vi "MotorControllerOpen.vi"(3 "error in":errorcluster, 4 "RefnumName":string, 5 "MotorConfig":T6={"CAN Address"=0, "Invert"=FALSE, "InvertSensor"=FALSE, "Unit Conversion Factor"=0.0, "Brake Mode"=enum."Override to Brake", "Reverse Limt Switch Mode"=enum."Disabled", "Forward Limt Swith Mode"=enum."Disabled", "PWM Channel"=enum."Invalid", "Motor Controller Type"=enum."Talon SRX", "Peak Current (A)"=0, "Continuous Current (A)"=0, "Peak Duration (ms)"=0, "Current Limit Enable"=FALSE}) -> (0 "error out":errorcluster, 2 "MotorControlDevRef":T1={"DeviceStatus"={"status"=FALSE, "code"=0, "source"=""}, "Type"=enum."PWM", "PWM"={"PWM Channel"=enum."Invalid", "DeadBand"={"Name"="", "maxPositivePwm"=0, "minPositivePwm"=0, "centerPwm"=0, "maxNegativePwm"=0, "minNegativePwm"=0, "angularRange"=0}}, "CAN"={"Device Number"=0, "SetOutput VI Ref"=variant(refnum<vi> refnum), "GetOutput VI Ref"=variant(refnum<vi> refnum), "Enable VI Ref"=variant(refnum<vi> refnum), "Disable VI Ref"=variant(refnum<vi> refnum), "Data"=variant}, "Invert"=FALSE, "DIO PWM"={"PWM \"Enable\" Channel"=enum."Invalid", "DIOChannel"=enum."Invalid", "PWM Rate"=0.0}})   [LabVIEW 2019, in "ArgosLib.lvlib"]
uses:
  ArgosLib.lvlib
  Config/ConfigComponents/TypeDefs/Config_Motor.ctl
  <vilib>/Rock Robotics/WPI/ThirdParty/Phoenix-LabVIEW/Motor Controller/Controls/CTRE_Phoenix_MotorControl_NeutralMode.ctl
  <vilib>/Rock Robotics/WPI/ThirdParty/Phoenix-LabVIEW/Motor Controller/Controls/CTRE_Phoenix_MotorControl_LimitSwitchNormal.ctl
  <vilib>/Rock Robotics/SystemInterfaces/DIO/FPGA_DIOPWMChannel.ctl
  Config/ConfigComponents/TypeDefs/Config_MotorCtrlType.ctl
  <vilib>/Rock Robotics/WPI/MotorControl/WPI_MotorControlDeviceRef.ctl
  <vilib>/Rock Robotics/WPI/MotorControl/WPI_MotorControlType.ctl
  <vilib>/Rock Robotics/WPI/PWM/WPI_PWMDeadband.ctl
  <vilib>/Rock Robotics/SystemInterfaces/DIO/FPGA_DIOChannel.ctl
  <vilib>/Rock Robotics/WPI/MotorControl/WPI_MotorControlOpen Talon.vi
  <vilib>/Playing With Fusion Inc/Playing With Fusion Lib for FRC/PWF_Venom_LabVIEW/PwF_Venom.lvlib
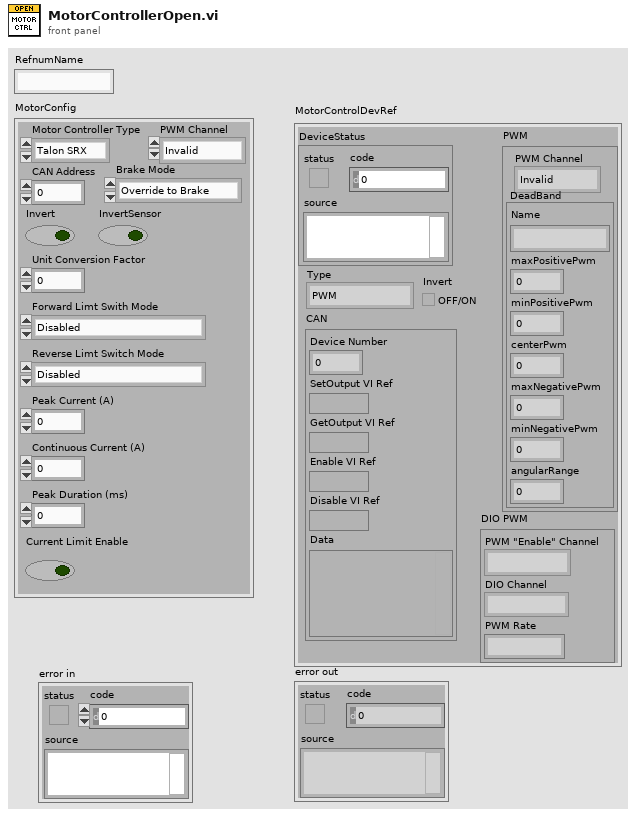
[diagram p1: front panel]
types:
  T1 = typedef "WPI_MotorControlDeviceRef.ctl" = cluster{"DeviceStatus":errorcluster, "Type":T2, "PWM":cluster{"PWM Channel":T3, "DeadBand":T4}, "CAN":cluster{"Device Number":u8, "SetOutput VI Ref":variant, "GetOutput VI Ref":variant, "Enable VI Ref":variant, "Disable VI Ref":variant, "Data":variant}, "Invert":bool, "DIO PWM":cluster{"PWM \"Enable\" Channel":T3, "DIOChannel":T5, "PWM Rate":dbl}}
  T2 = typedef "WPI_MotorControlType.ctl" = enum16{"PWM", "CAN", "DIO PWM"}
  T3 = typedef "FPGA_DIOPWMChannel.ctl" = enum8{"PWM 0", "PWM 1", "PWM 2", "PWM 3", "PWM 4", "PWM 5", "PWM 6", "PWM 7", "PWM 8", "PWM 9", "PWM MXP 0", "PWM MXP 1", "PWM MXP 2", "PWM MXP 3", "PWM MXP 4", "PWM MXP 5", "PWM MXP 6", "PWM MXP 7", "PWM MXP 8", "PWM MXP 9", "Invalid"}
  T4 = typedef "WPI_PWMDeadband.ctl" = cluster{"Name":string, "maxPositivePwm":i32, "minPositivePwm":i32, "centerPwm":i32, "maxNegativePwm":i32, "minNegativePwm":i32, "angularRange":u16}
  T5 = typedef "FPGA_DIOChannel.ctl" = enum8{"DIO 0", "DIO 1", "DIO 2", "DIO 3", "DIO 4", "DIO 5", "DIO 6", "DIO 7", "DIO 8", "DIO 9", "DIO MXP 0", "DIO MXP 1", "DIO MXP 2", "DIO MXP 3", "DIO MXP 4", "DIO MXP 5", "DIO MXP 6", "DIO MXP 7", "DIO MXP 8", "DIO MXP 9", "DIO MXP 10", "DIO MXP 11", "DIO MXP 12", "DIO MXP 13", "DIO MXP 14", "DIO MXP 15", "SPI Port CS1", "SPI Port CS2", "SPI Port CS3", "SPI Port MISO", "SPI Port MOSI", "Invalid"}
  T6 = typedef "ArgosLib.lvlib/Config_Motor.ctl" = cluster{"CAN Address":u8, "Invert":bool, "InvertSensor":bool, "Unit Conversion Factor":dbl, "Brake Mode":T7, "Reverse Limt Switch Mode":T8, "Forward Limt Swith Mode":T8, "PWM Channel":T3, "Motor Controller Type":T9, "Peak Current (A)":i32, "Continuous Current (A)":i32, "Peak Duration (ms)":i32, "Current Limit Enable":bool}
  T7 = typedef "CTRE_Phoenix_MotorControl_NeutralMode.ctl" = enum8{"EEPROMSetting", "Override to Coast", "Override to Brake"}
  T8 = typedef "CTRE_Phoenix_MotorControl_LimitSwitchNormal.ctl" = enum16{"Normally Open", "Normally Closed", "Disabled"}
  T9 = typedef "ArgosLib.lvlib/Config_MotorCtrlType.ctl" = enum16{"Disabled", "Talon SRX", "Talon SR", "Venom", "Spark MAX", "Falcon FX"}
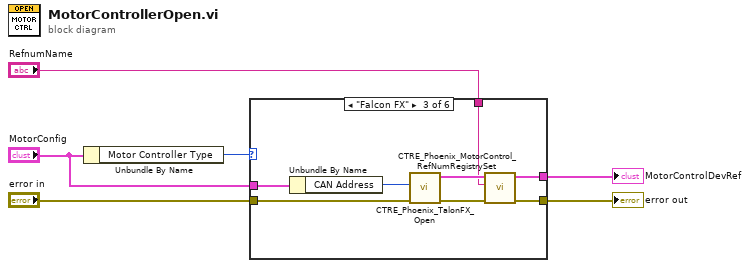
[diagram p0: block diagram]
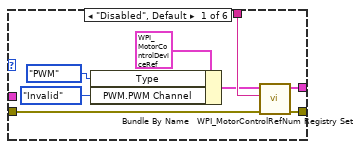
[diagram p2: hidden frame]
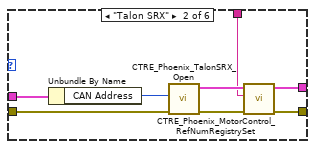
[diagram p3: hidden frame]
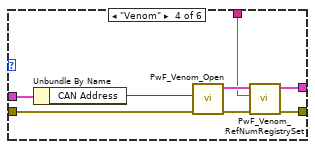
[diagram p4: hidden frame]
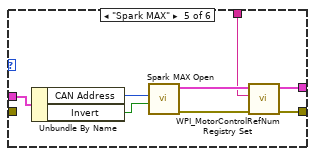
[diagram p5: hidden frame]
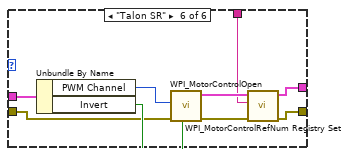
[diagram p6: hidden frame]
diagram:
  n1 = Unbundle By Name("MotorConfig") -> ("Motor Controller Type"=w6:T9)
  n2 = case shown="\"Falcon FX\"" w6 {
    tunnel: "MotorConfig" -> [_ w22 w30 w33 w46 w55]
    tunnel: "error in" -> [w8 w20 w28 w31 _ w52]
    tunnel: "RefnumName" -> [w12 w17 w25 w34 w41 w49]
    tunnel: [w13 w16 w24 w36 w42 w48] -> w2
    tunnel: [w14 w15 w23 w35 w44 w47] -> w1
    frame "Disabled", Default {
      n3 = Bundle By Name(cluster=T1 {"DeviceStatus"={"status"=FALSE, "code"=0, "source"=""}, "Type"=enum."PWM", "PWM"={"PWM Channel"=enum."Invalid", "DeadBand"={"Name"="", "maxPositivePwm"=0, "minPositivePwm"=0, "centerPwm"=0, "maxNegativePwm"=0, "minNegativePwm"=0, "angularRange"=0}}, "CAN"={"Device Number"=0, "SetOutput VI Ref"=variant(refnum<vi> refnum), "GetOutput VI Ref"=variant(refnum<vi> refnum), "Enable VI Ref"=variant(refnum<vi> refnum), "Disable VI Ref"=variant(refnum<vi> refnum), "Data"=variant}, "Invert"=FALSE, "DIO PWM"={"PWM \"Enable\" Channel"=enum."Invalid", "DIOChannel"=enum."Invalid", "PWM Rate"=0.0}} ("MotorControlDeviceRef"), "Type"=WPI_MotorControlType."PWM", "PWM.PWM Channel"=FPGA_DIOPWMChannel."Invalid") -> (w7:T1)
      n4 = call <vilib>:"WPI_MotorControlRefNum Registry Set.vi"("error in (no error)"=w8, "refnum name"=w12, "MotorControlDevRef"=w7) -> ("error out"=w14:errorcluster, "MotorControlDevRef"=w13:T1)  [unwired: 7 in]
    }
    frame "Talon SRX" {
      n5 = Unbundle By Name(w22) -> ("CAN Address"=w21:u8)
      n6 = call <vilib>:"CTRE_Phoenix_TalonSRX_Open.vi"("error in"=w20, "Device Number"=w21) -> ("error out"=w19:errorcluster, "CAN Talon SRX Ref"=w18:T1)  [unwired: 8 in]
      n7 = call <vilib>:"CTRE_Phoenix_MotorControl_RefNumRegistrySet.vi"("error in (no error)"=w19, "refnum name"=w17, "PhoenixMotorControlDevRef"=w18) -> ("error out"=w15:errorcluster, "PhoenixMotorControlDevRef"=w16:T1)  [unwired: 7 in]
    }
    frame "Falcon FX" {
      n8 = Unbundle By Name(w30) -> ("CAN Address"=w29:u8)
      n9 = call <vilib>:"CTRE_Phoenix_TalonFX_Open.vi"("error in"=w28, "Device Number"=w29) -> ("error out"=w27:errorcluster, "CAN Talon SRX Ref"=w26:T1)  [unwired: 8 in]
      n10 = call <vilib>:"CTRE_Phoenix_MotorControl_RefNumRegistrySet.vi"("error in (no error)"=w27, "refnum name"=w25, "PhoenixMotorControlDevRef"=w26) -> ("error out"=w23:errorcluster, "PhoenixMotorControlDevRef"=w24:T1)  [unwired: 7 in]
    }
    frame "Venom" {
      n11 = Unbundle By Name(w33) -> ("CAN Address"=w32:u8)
      n12 = call <vilib>:"PwF_Venom_Open.vi"("error in"=w31, "Device Number"=w32) -> ("error out"=w38:errorcluster, "Venom Ref"=w37:T1)  [unwired: 8 in]
      n13 = call <vilib>:"PwF_Venom_RefNumRegistrySet.vi"("error in (no error)"=w38, "refnum name"=w34, "PwFVenomDevRefIn"=w37) -> ("error out"=w35:errorcluster, "PwFVenomDevRefOut"=w36:T1)  [unwired: 7 in]
    }
    frame "Spark MAX" {
      n14 = Unbundle By Name(w46) -> ("CAN Address"=w45:u8, "Invert"=w39:bool)
      n15 = call <vilib>:"Spark MAX Open.vi"("Invert"=w39, "Device Number"=w45) -> ("error out"=w40:errorcluster, "MotorControlDeviceRef"=w43:T1)  [unwired: 8 in]
      n16 = call <vilib>:"WPI_MotorControlRefNum Registry Set.vi"("error in (no error)"=w40, "refnum name"=w41, "MotorControlDevRef"=w43) -> ("error out"=w44:errorcluster, "MotorControlDevRef"=w42:T1)  [unwired: 7 in]
    }
    frame "Talon SR" {
      n17 = Unbundle By Name(w55) -> ("PWM Channel"=w53:T3, "Invert"=w54:bool)
      n18 = call-poly <vilib>:"WPI_MotorControlOpen.vi"("Invert"=w54, "error in (no error)"=w52, "PWM Channel"=w53) -> ("error out"=w50:errorcluster, "MotorControlDeviceRef"=w51:T1)  [unwired: 7 in]
      n19 = call <vilib>:"WPI_MotorControlRefNum Registry Set.vi"("error in (no error)"=w50, "refnum name"=w49, "MotorControlDevRef"=w51) -> ("error out"=w47:errorcluster, "MotorControlDevRef"=w48:T1)  [unwired: 7 in]
    }
  }
  "MotorControlDevRef" <- w2
  "error out" <- w1
